vi "Esophageal_GenerateSubfolders.vi"(8 "error in":errorcluster, 11 "Patient Data Folder":path=path "C:/Users/ABGS_/Desktop/ABGS_RT_HRME Frames/TestFolders") -> (0 "error out":errorcluster, 2 "HRME Scores":path, 3 "QC Pass Path":path, 4 "Representative Images":path)   [LabVIEW 2021]
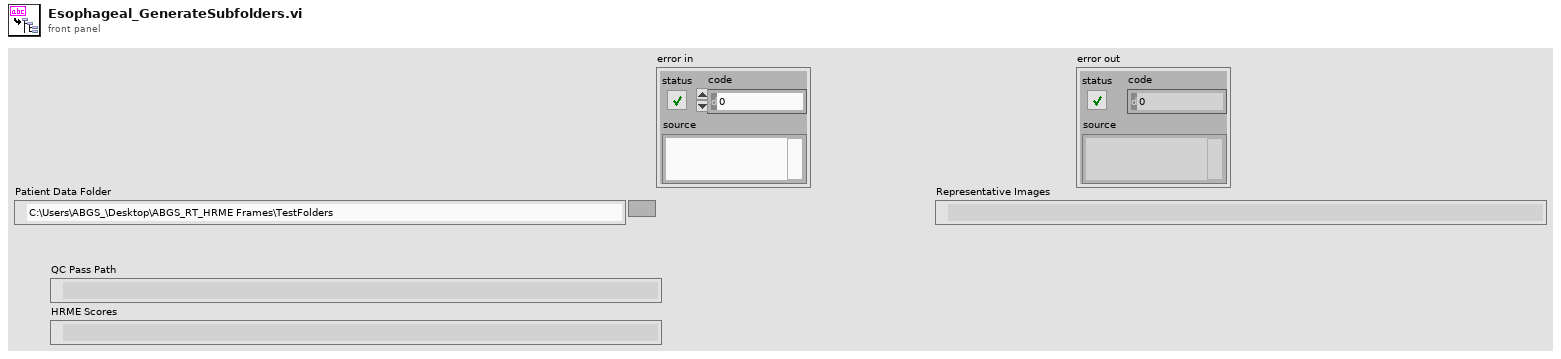
[diagram p1: front panel]
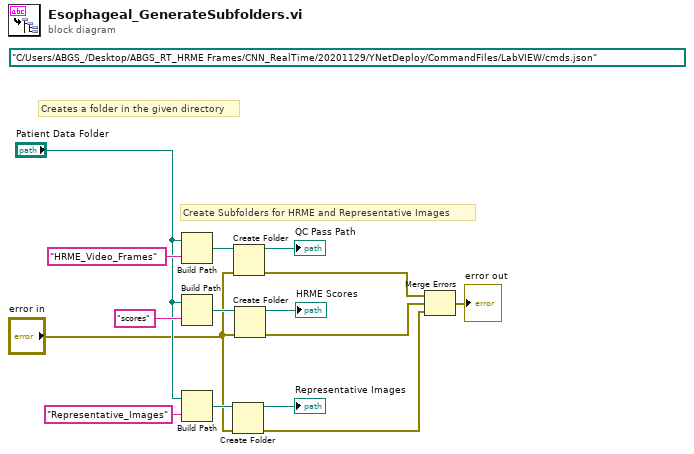
[diagram p0: block diagram]
diagram:
  (unwired) path "C:/Users/ABGS_/Desktop/ABGS_RT_HRME Frames/CNN_RealTime/20201129/YNetDeploy/CommandFiles/LabVIEW/cmds.json" ("Command File Location")
  # "Create Subfolders for HRME and Representative Images"
  # "Creates a folder in the given directory"
  n1 = Build Path(base path="Patient Data Folder", name or relative path="HRME_Video_Frames") -> (appended path=w13:path)
  n2 = Build Path(base path="Patient Data Folder", name or relative path="scores") -> (appended path=w12:path)
  n3 = Build Path(base path="Patient Data Folder", name or relative path="Representative_Images") -> (appended path=w5:path)
  n4 = Create Folder(path (use dialog)=w5, error in="error in") -> (created path=→"Representative Images":path, error out=w1:errorcluster)  [unwired: 1 in, 1 out]
  n5 = Create Folder(path (use dialog)=w13, error in="error in") -> (created path=→"QC Pass Path":path, error out=w8:errorcluster)  [unwired: 1 in, 1 out]
  n6 = Create Folder(path (use dialog)=w12, error in="error in") -> (created path=→"HRME Scores":path, error out=w7:errorcluster)  [unwired: 1 in, 1 out]
  n7 = Merge Errors(w8, w7, w1) -> (→"error out":errorcluster)
